vi "Wait_PTB.vi"(0 "Data Task in":refnum<k21>, 5 "data task error in":errorcluster, 7 "#DAQ outputs (1-13)":i32, 9 "PS VISA in":refnum<visa-resource-name>, 11 "PS error in":errorcluster caption="PS error in (no error)", 12 "Wait Filepath":path=path "C:/Users/ga11/Desktop/VI/results/3PtestChrgRest.lvm" caption="Filename", 13 "Wait time":dbl) -> (4 "data task out":refnum<k21>, 6 "data task error out":errorcluster, 10 "PS Visa Out":refnum<visa-resource-name>, 15 "PS error out":errorcluster)   [LabVIEW 2020]
uses:
  Parallel-Current-Analysis-Platform-PCAP/parallel_testbed/IT-M3400/IT-M3400.lvlib
panel:
  out "WaitElapsed Time (s)":i32 caption="Elapsed Time (s)"
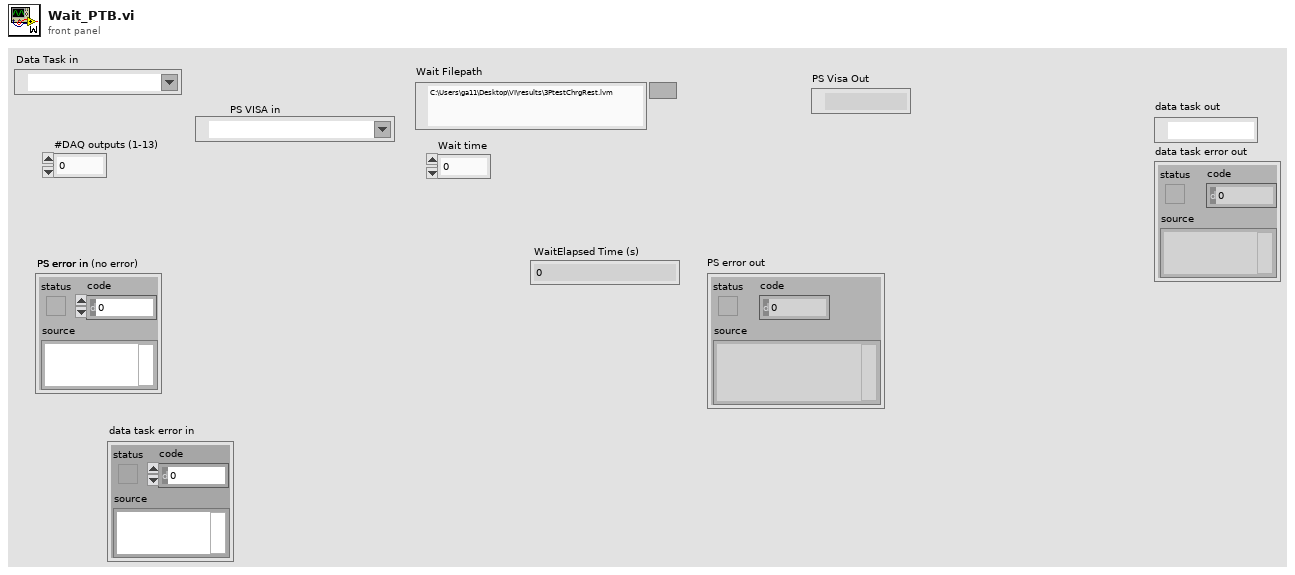
[diagram p1: front panel]
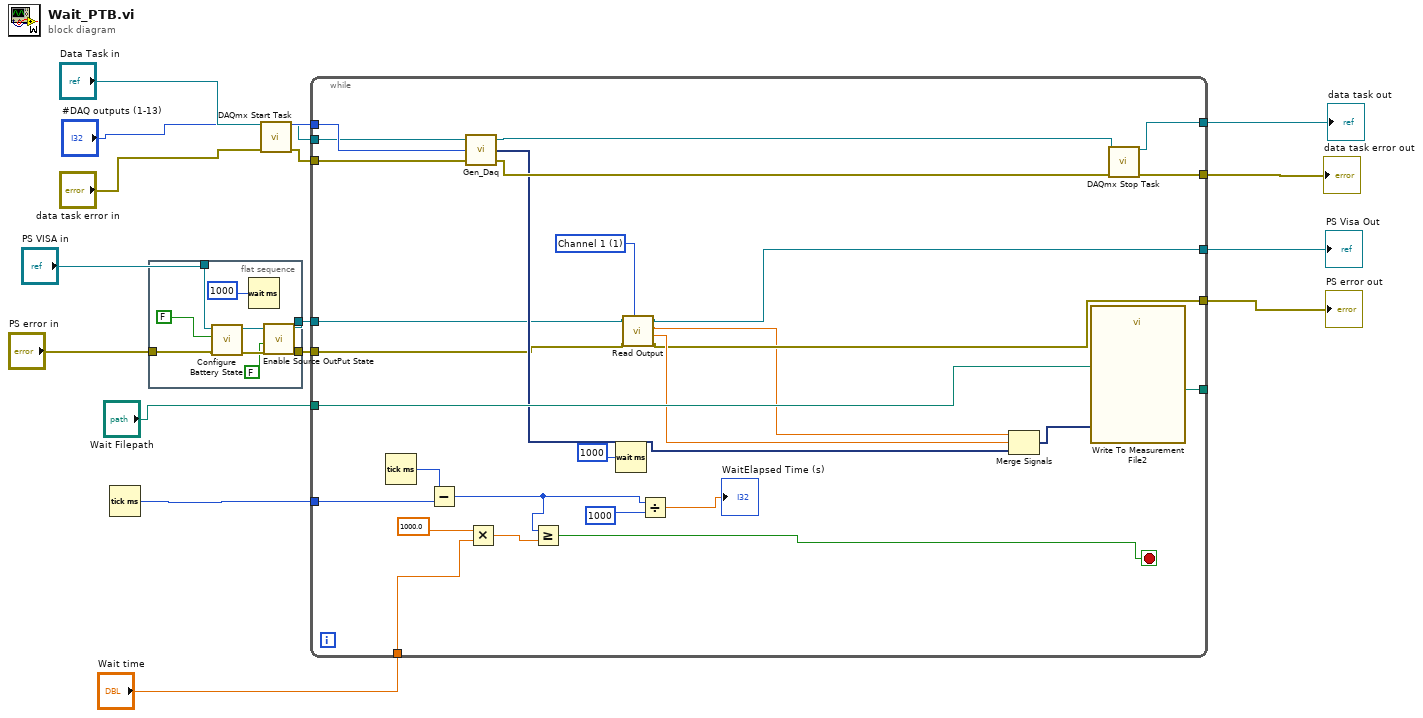
[diagram p0: block diagram]
diagram:
  n1 = Tick Count (ms)() -> (millisecond timer value=w15:u32)
  n2 = flat-sequence {
    tunnel: "PS VISA in" -> [w25]
    tunnel: "PS error in" -> [w24]
    tunnel: [w20] -> w2
    tunnel: [w19] -> w1
    frame #0 {
      n3 = call "Configure Battery State.vi"("error in"=w24, "State"=FALSE, "VISA resource name"=w25) -> ("error out"=w21:errorcluster, "VISA resource name out"=w22:refnum<visa-resource-name>)  [unwired: 7 in]
      n4 = Wait (ms)(milliseconds to wait=1000) -> ()  [unwired: 1 out]
      n5 = call "Enable Source OutPut State.vi"("error in"=w21, "State"=FALSE, "VISA resource name"=w22) -> ("error out"=w20:errorcluster, "VISA resource name out"=w19:refnum<visa-resource-name>)  [unwired: 7 in]
    }
  }
  n6 = call <vilib>:"DAQmx Start Task.vi"("task/channels in"="Data Task in", "error in"="data task error in") -> ("task out"=w6:refnum<k21>, "error out"=w5:errorcluster)  [unwired: 12 in]
  n7 = while {
    tunnel: "Wait time" -> [w50]
    tunnel: [w47] -> _
    tunnel: w15 -> [w46]
    tunnel: "Wait Filepath" -> [w45]
    tunnel: [w29] -> w13
    tunnel: [w28] -> w12
    tunnel: "#DAQ outputs (1-13)" -> [w39]
    tunnel: w6 -> [w38]
    tunnel: w5 -> [w37]
    tunnel: [w36] -> w8
    tunnel: [w35] -> w7
    tunnel: w1 -> [w32]
    tunnel: w2 -> [w31]
    stop <- w51 stop-if-true
    w27 = 1 items=["Channel 1"=1, "Channel 2"=2, "Channel 3"=3, "Channel 4"=4, "Channel 5"=5, "Channel 6"=6, "Channel 7"=7, "Channel 8"=8, "Channel 8"=9, "Channel 10"=10, "Channel 11"=11, "Channel 12"=12, "Channel 13"=13, "Channel 14"=14, "Channel 15"=15, "Channel 16"=16] ("Channel")
    n8 = Tick Count (ms)() -> (millisecond timer value=w52:u32)
    n9 = Subtract(x=w52, y=w46) -> (x-y=w33:u32)
    n10 = call "Gen_Daq.vi"("error in"=w37, "#DAQ outputs (1-13)"=w39, "task/channels in"=w38) -> ("error out"=w40:errorcluster, "DaQ_output"=w34:dynamicdata, "task out"=w41:refnum<k21>)
    n11 = Multiply(x=1000.0, y=w50) -> (x*y=w48:dbl)
    n12 = Greater Or Equal?(x=w33, y=w48) -> (x >= y?=w51:bool)
    n13 = Wait (ms)(milliseconds to wait=1000) -> ()  [unwired: 1 out]
    n14 = call "Read Output.vi"("Channel"=w27, "error in"=w31, "VISA resource name"=w32) -> ("error out"=w28:errorcluster, "Read Current(A)"=w30:dbl, "Read Voltage(V)"=w26:dbl, "VISA resource name out"=w29:refnum<visa-resource-name>)  [unwired: 5 in]
    n15 = Divide(x=w33, y=1000) -> (x/y=→"WaitElapsed Time (s)":dbl)
    n16 = Merge Signals "Merge Signals"(w26, w30, w34) -> (w42:dynamicdata)
    n17 = call "Write To Measurement File2"("Signals"=w42, "Filename"=w45) -> ("Filename Out"=w47:path)  [unwired: 15 in, 2 out]
    n18 = call <vilib>:"DAQmx Stop Task.vi"("task/channels in"=w41, "error in"=w40) -> ("task out"=w36:refnum<k21>, "error out"=w35:errorcluster)  [unwired: 12 in]
  }
  "PS Visa Out" <- w13
  "PS error out" <- w12
  "data task out" <- w8
  "data task error out" <- w7
